vi "CheckXYPlaneCoords (SubVI).vi"(4 "Yhigh":dbl=150.0 format="%#_13g", 5 "Xhigh":dbl=750.0 format="%#_13g", 6 "Ylow":dbl=-150.0 format="%#_13g", 7 "Xlow":dbl=-750.0 format="%#_13g", 10 "Jog Distance":T1, 11 "Go to Coordinates":T1) -> (3 "Pass record":bool[](array[boolean]))   [LabVIEW 2016]
panel:
  # "-x, +x, -y, +y"
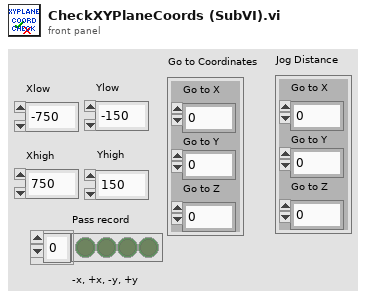
[diagram p1: front panel]
types:
  T1 = cluster{"Go to X":dbl, "Go to Y":dbl, "Go to Z":dbl}
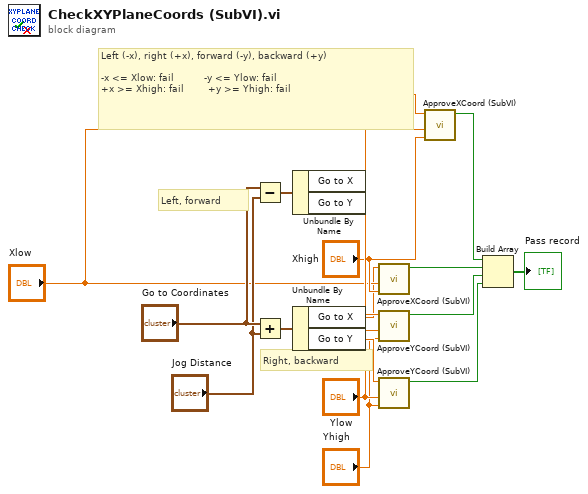
[diagram p0: block diagram]
diagram:
  # "Left, forward"
  # "Right, backward"
  # "Left (-x), right (+x), forward (-y), backward (+y)\n\n-x <= Xlow: fail          -y <= Ylow: fail\n+x >= Xhigh: fail        +y >= Yhigh: fail"
  n1 = Subtract(x="Go to Coordinates", y="Jog Distance") -> (x-y=w15:T1)
  n2 = Add(x="Go to Coordinates", y="Jog Distance") -> (x+y=w14:T1)
  n3 = Unbundle By Name(w15) -> ("Go to X"=w11:dbl, "Go to Y"=w12:dbl)
  n4 = Unbundle By Name(w14) -> ("Go to X"=w8:dbl, "Go to Y"=w13:dbl)
  n5 = call "ApproveXCoord (SubVI).vi"("Xhigh"="Xhigh", "Xlow"="Xlow", "Go to X"=w8) -> ("Pass X?"=w1:bool)  [unwired: 8 in]
  n6 = call "ApproveYCoord (SubVI).vi"("Yhigh"="Yhigh", "Ylow"="Ylow", "Go to Y"=w12) -> ("Pass Y?"=w2:bool)  [unwired: 8 in]
  n7 = call "ApproveYCoord (SubVI).vi"("Yhigh"="Yhigh", "Ylow"="Ylow", "Go to Y"=w13) -> ("Pass Y?"=w4:bool)  [unwired: 8 in]
  n8 = call "ApproveXCoord (SubVI).vi"("Xhigh"="Xhigh", "Xlow"="Xlow", "Go to X"=w11) -> ("Pass X?"=w5:bool)  [unwired: 8 in]
  n9 = Build Array(w5, w1, w2, w4) -> (→"Pass record":bool[])
